vi "Polynomial Eigenvalues and Vectors.vi"   [LabVIEW 2010, in "NI_AALPro.lvlib"]
doc: "Solves the polynomial eigenvalue problem. Wire data to the <B>Input Matrices</B> input to determine the polymorphic instance to use or manually select the instance."
uses:
  NI_AALPro.lvlib
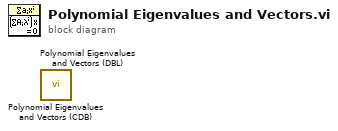
[diagram p0: block diagram]
diagram:
  n1 = call "Polynomial Eigenvalues and Vectors (CDB).vi"() -> ()  [unwired: 9 in, 3 out]
  n2 = call "Polynomial Eigenvalues and Vectors (DBL).vi"() -> ()  [unwired: 9 in, 3 out]
